vi "GetSignals.vi"(8 "Error in":errorcluster, 10 "FirstSignalsOnly":bool=TRUE, 11 "Devices":refnum<k24>[](array[refnum])) -> (0 "Error out":errorcluster, 2 "DevInfo":T1(array[cluster]), 3 "DevicesAndSignals":T2)   [LabVIEW 2016]
doc: "Delivers (all) signals of the given devices.\n\nDevices: Devices from which to deliver the signals\nFirstSignalsOnly: Set to true (default) if you only want the get the respective first signals of each channel (QuantumX devices return 2 signals per channel if FirstSignalsOnly is set to false).\n\nDevicesAndSignals: Cluster consisting of an array of devices and an array of all signals of the given devices"
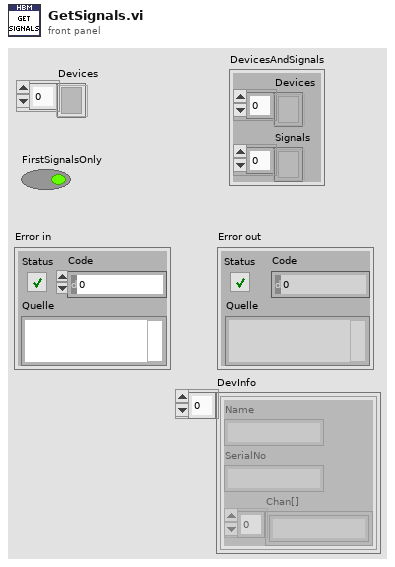
[diagram p1: front panel]
types:
  T1 = cluster{"Name":string, "SerialNo":string, "Chan[]":string[]}[]
  T2 = cluster{"Devices":refnum<k24>[], "Signals":refnum<k24>[]}
  T3 = cluster{"Name":string, "SerialNo":string, string[]}
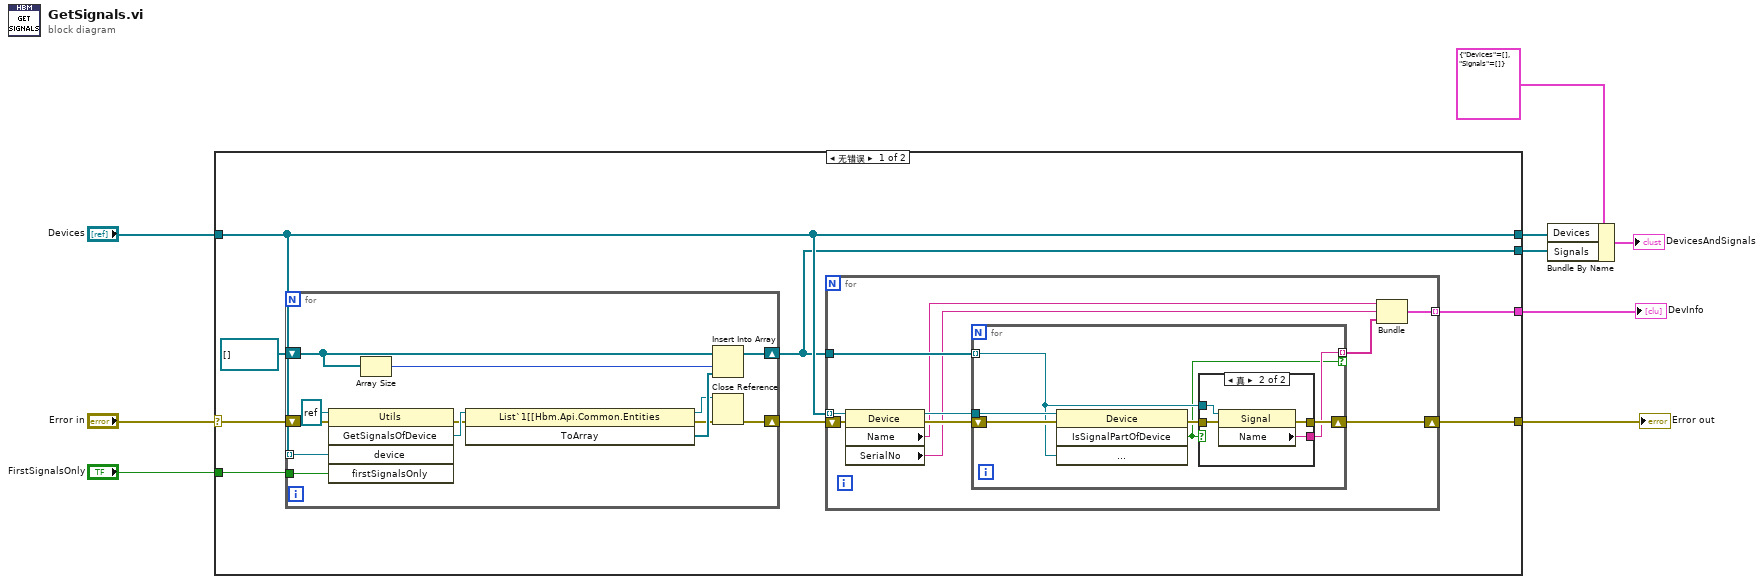
[diagram p0: block diagram]
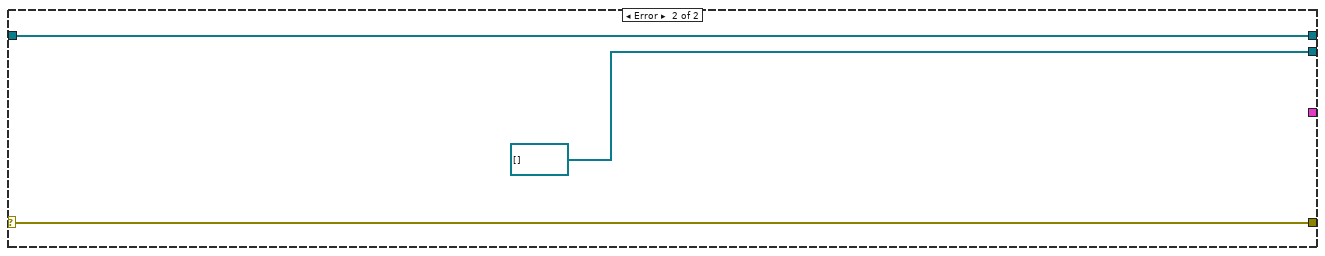
[diagram p3: hidden frame]
diagram:
  n1 = case shown="无错误" "Error in" {
    selector: "Error in" -> [w16 w54]
    tunnel: [w15 w54] -> w9
    tunnel: [w11 refnum<k24>[] [] ("ToArray")] -> w3
    tunnel: "Devices" -> [w12 w52]
    tunnel: [w12 w52] -> w4
    tunnel: "FirstSignalsOnly" -> [w13 _]
    tunnel: [w10 _] -> w1
    frame No Error {
      n2 = for {
        shift-right: [w51] -> w11
        shift-left: refnum<k24>[] [] -> [w50]
        shift-right: [w41] -> w15
        shift-left: w16 -> [w46]
        tunnel: w12 -> [w45] mode=indexing
        tunnel: w13 -> [w44]
        n3 = invoke on="Methodenknoten" class="Utils" method="GetSignalsOfDevice"(reference=refnum<k24> refnum, error in=w46, "device"=w45, "firstSignalsOnly"=w44) -> (error out=w47:errorcluster, "GetSignalsOfDevice"=w48:refnum<k24>)  [unwired: 1 in, 3 out]
        n4 = Array Size(array=w50) -> (size(s)=w49:i32)
        n5 = invoke on="Methodenknoten" class="List`1[[Hbm.Api.Common.Entities" method="ToArray"(reference=w48, error in=w47) -> (reference out=w40:refnum<k24>, error out=w42:errorcluster, "ToArray"=w43:refnum<k24>[])  [unwired: 1 in]
        n6 = Insert Into Array(array=w50, index=w49, new element=w43) -> (w51:refnum<k24>[])
        n7 = Close Reference(reference=w40, error in (no error)=w42) -> (error out=w41:errorcluster)
      }
      n8 = for {
        tunnel: w12 -> [w24] mode=indexing
        tunnel: w11 -> [w26]
        shift-right: [w25] -> _
        shift-left: _ -> [w22]
        tunnel: [w17] -> w10 mode=indexing
        n9 = property on="Eigenschaftsknoten" class="Device"(reference=w24, error in=w22) -> (reference out=w23:refnum<k24>, error out=w21:errorcluster, "Name"=w20:string, "SerialNo"=w19:string)
        n10 = for {
          tunnel: w23 -> [w33]
          tunnel: w26 -> [w30] mode=indexing
          shift-right: [w29] -> w25
          shift-left: w21 -> [w32]
          tunnel: [w28] -> w18 mode=indexing if=w27
          n11 = invoke on="Methodenknoten" class="Device" method="IsSignalPartOfDevice"(reference=w33, error in=w32, "signalToCheck"=w30) -> (error out=w31:errorcluster, "IsSignalPartOfDevice"=w27:bool)  [unwired: 1 in, 2 out]
          n12 = case shown="真" w27 {
            tunnel: w31 -> [w34 w37]
            tunnel: w30 -> [_ w38]
            tunnel: [w34 w36] -> w29
            tunnel: [_ w35] -> w28
            frame False {
            }
            frame True {
              n13 = property on="Eigenschaftsknoten" class="Signal"(reference=w38, error in=w37) -> (error out=w36:errorcluster, "Name"=w35:string)  [unwired: 1 out]
            }
          }
        }
        n14 = Bundle("Name"=w20, "SerialNo"=w19, w18) -> (w17:T3)  [unwired: 1 in]
      }
    }
    frame Error {
    }
  }
  "Error out" <- w9
  "DevInfo" <- w1
  n15 = Bundle By Name(cluster=T2 {"Devices"=[], "Signals"=[]} ("DevicesAndSignals"), "Devices"=w4, "Signals"=w3) -> (→"DevicesAndSignals":T2)
